vi "扫码查询B.vi"(9 "2D_Code":string) -> (1 "Match":i32, 3 "Data":string[][](array[string]))   [LabVIEW 2014]
panel:
  out "error out":errorcluster
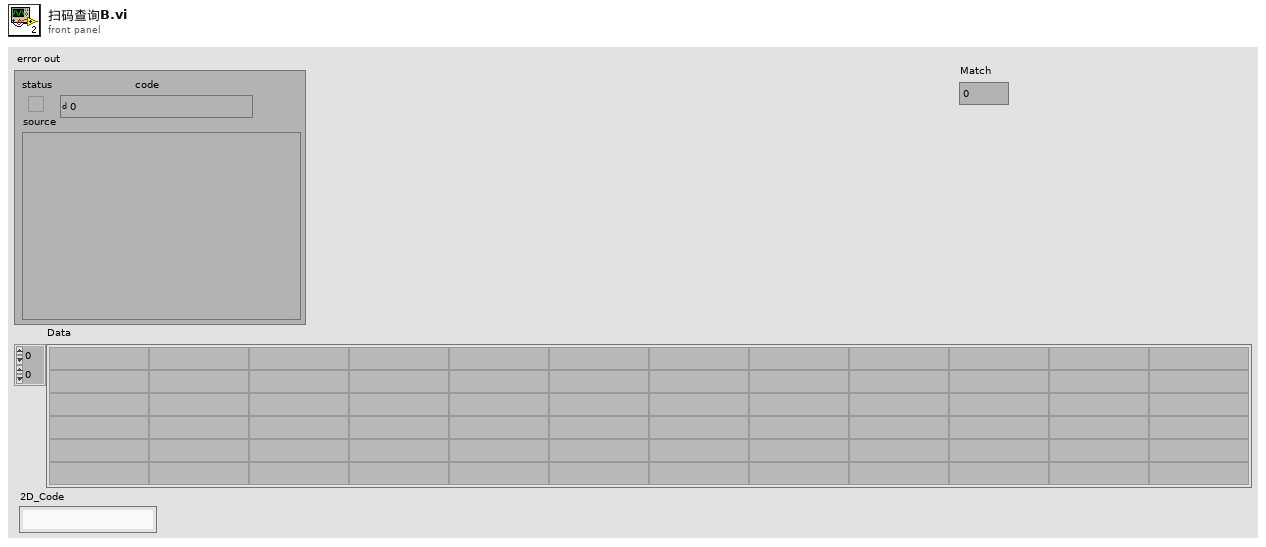
[diagram p1: front panel]
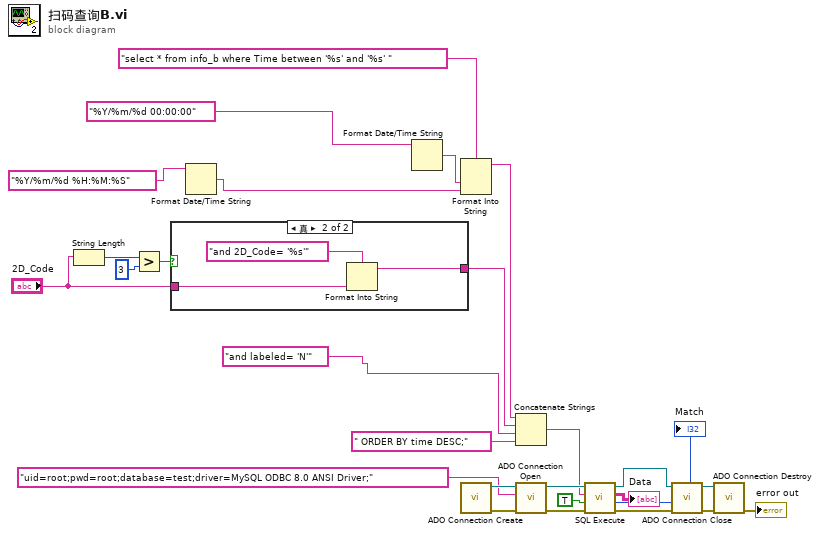
[diagram p0: block diagram]
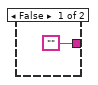
[diagram p2: hidden frame]
diagram:
  n1 = String Length(string="2D_Code") -> (length=w6:i32)
  n2 = Greater?(x=w6, y=3) -> (0:w4:bool)
  n3 = case shown="真" w4 {
    tunnel: ["" w31] -> w9
    tunnel: "2D_Code" -> [_ w29]
    frame False {
    }
    frame True {
      n4 = Format Into String(format string="and 2D_Code= '%s'" ("字符串"), w29) -> (resulting string=w31:string)  [unwired: 2 in, 1 out]
    }
  }
  n5 = Format Date/Time String(time format string (%c)="%Y/%m/%d %H:%M:%S" ("时间格式字符串(%c)")) -> (date/time string=w12:string)  [unwired: 2 in]
  n6 = Format Date/Time String(time format string (%c)="%Y/%m/%d 00:00:00" ("时间格式字符串(%c)")) -> (date/time string=w13:string)  [unwired: 2 in]
  n7 = Format Into String(format string="select * from info_b where Time between '%s' and '%s' " ("Command Text"), w13, w12) -> (resulting string=w11:string)  [unwired: 2 in, 1 out]
  n8 = call "ADO Connection Create.vi"() -> ("error out"=w26:errorcluster, "ADODB._Connection Out"=w27:refnum<k7>)  [unwired: 10 in]
  n9 = Concatenate Strings(w11, w9, "and labeled= 'N'" ("字符串"), " ORDER BY time DESC;" ("字符串")) -> (w8:string)
  n10 = call "ADO Connection Open.vi"("error in (no error)"=w26, "ConnectionString"="uid=root;pwd=root;database=test;driver=MySQL ODBC 8.0 ANSI Driver;", "ADODB._Connection In"=w27) -> ("error out"=w24:errorcluster, "ADODB._Connection Out"=w25:refnum<k7>)  [unwired: 7 in]
  n11 = call "SQL Execute.vi"("error in (no error)"=w24, "Return Data (T)"=TRUE, "Command Text"=w8, "ADODB._Connection In"=w25) -> ("error out"=w22:errorcluster, "Rows Fetched"=→"Match":i32, "Data"=→"Data":string[][], "ADODB._Connection Out"=w23:refnum<k7>)  [unwired: 4 in]
  n12 = call "ADO Connection Close.vi"("error in (no error)"=w22, "ADODB._Connection In"=w23) -> ("error out"=w20:errorcluster, "ADODB._Connection Out"=w21:refnum<k7>)  [unwired: 8 in]
  n13 = call "ADO Connection Destroy.vi"("error in (no error)"=w20, "ADODB._Connection In"=w21) -> ("error out"=→"error out":errorcluster)  [unwired: 9 in]
